vi "Shortest Distance Absolute.vi"(10 "current":dbl(knob) scale=0.0..360.0, 11 "target":dbl(knob) scale=0.0..360.0) -> (3 "shortest angle":dbl)   [LabVIEW 2014]
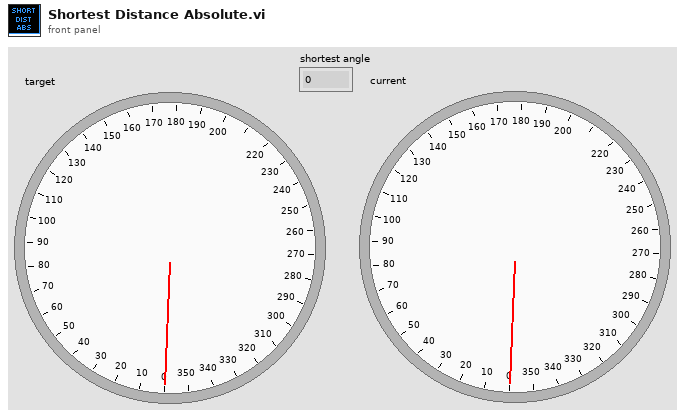
[diagram p1: front panel]
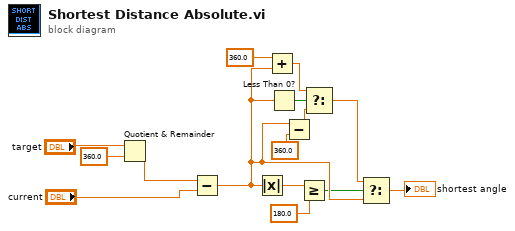
[diagram p0: block diagram]
diagram:
  n1 = Quotient & Remainder(x="target", y=360.0) -> (x-y*floor(x/y)=w2:dbl)  [unwired: 1 out]
  n2 = Subtract(x=w2, y="current") -> (x-y=w15:dbl)
  n3 = Absolute Value(x=w15) -> (abs(x)=w6:dbl)
  n4 = Add(x=360.0, y=w15) -> (x+y=w12:dbl)
  n5 = Less Than 0?(x=w15) -> (x < 0?=w10:bool)
  n6 = Subtract(x=w15, y=360.0 ("x")) -> (x-y=w11:dbl)
  n7 = Greater Or Equal?(x=w6, y=180.0) -> (x >= y?=w8:bool)
  n8 = Select(t=w12, s=w10, f=w11) -> (s? t:f=w9:dbl)
  n9 = Select(t=w9, s=w8, f=w15) -> (s? t:f=→"shortest angle":dbl)
